vi "Get filepath.vi"(8 "error in (no error)":errorcluster, 11 "DAQOrcaFlash in":refnum<class "DAQOrcaFlash.lvclass">) -> (0 "error out":errorcluster, 2 "full storage path":path, 3 "DAQOrcaFlash out":refnum<class "DAQOrcaFlash.lvclass">)   [LabVIEW 2012, in "DAQOrcaFlash.lvclass"]
uses:
  DAQOrcaFlash.lvclass
  DAQOrcaFlash.lvclass/DAQOrcaFlash.ctl
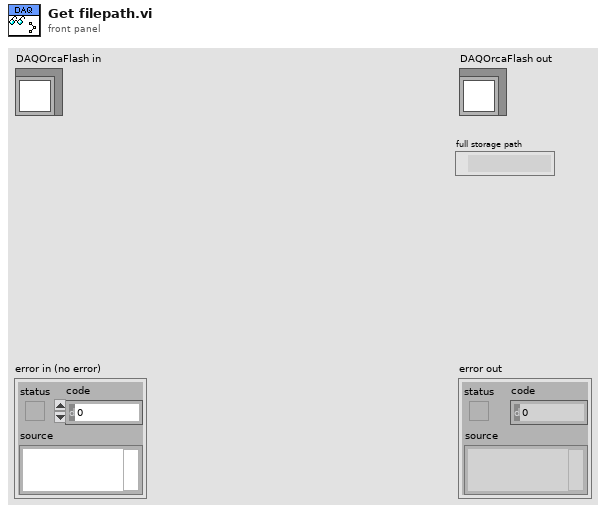
[diagram p1: front panel]
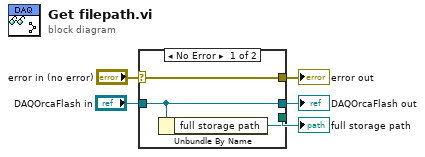
[diagram p0: block diagram]
diagram:
  n1 = case shown="No Error" "error in (no error)" {
    selector: "error in (no error)" -> [w8 w10]
    tunnel: [w8 w10] -> w4
    tunnel: [w7 w9] -> w2
    tunnel: "DAQOrcaFlash in" -> [w7 w9]
    tunnel: [w6 _] -> w1
    frame No Error {
      n2 = Unbundle By Name(w7) -> ("full storage path"=w6:path)
    }
    frame Error {
    }
  }
  "error out" <- w4
  "DAQOrcaFlash out" <- w2
  "full storage path" <- w1
